vi "myRIO__TCP_constants_byteRange_messageType_start.vi"() -> (2 "output_Start_byte":u8=83, 3 "output_Start_char":string="S")   [LabVIEW 2014]
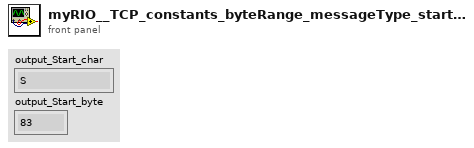
[diagram p1: front panel]
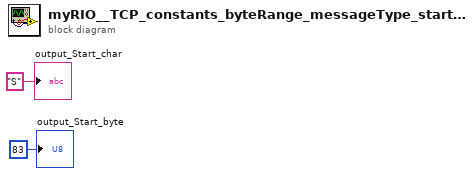
[diagram p0: block diagram]
diagram:
  "output_Start_char" <- "S"
  "output_Start_byte" <- u8 83
